vi "Log Trace.vi"(8 "error in (no error)":errorcluster, 10 "Trace.lvclass":refnum<class "Trace.lvclass">, 11 "Tracer in":refnum<class "Tracer.lvclass">) -> (0 "error out":errorcluster, 2 "TraceMessage Out":refnum<class "Trace.lvclass">, 3 "Tracer out":refnum<class "Tracer.lvclass">)   [LabVIEW 2013, in "Tracer.lvclass"]
uses:
  Tracer.lvclass
  TraceMessage/Trace.lvclass
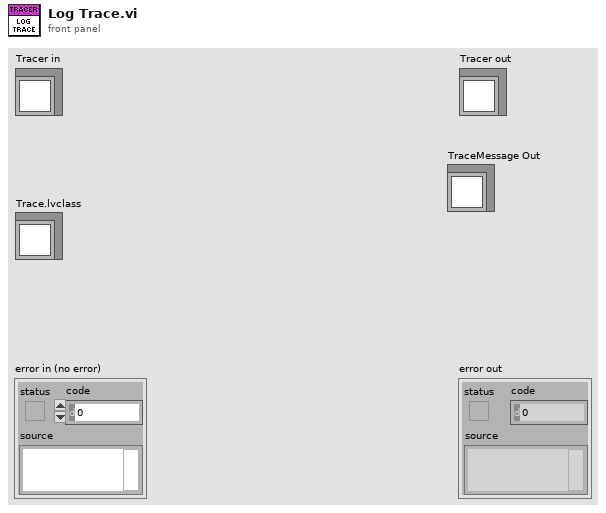
[diagram p1: front panel]
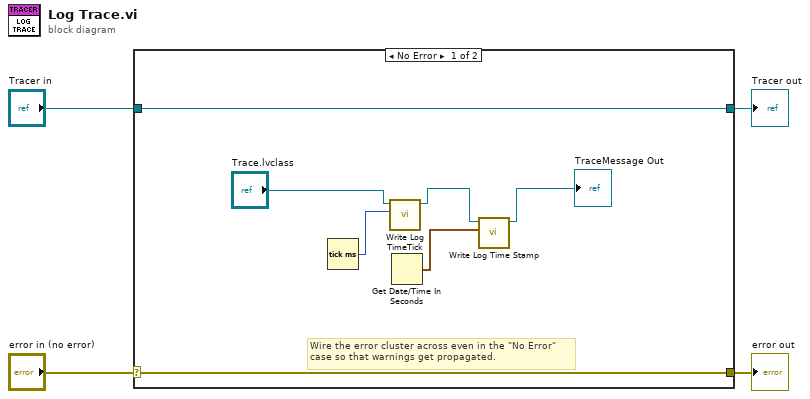
[diagram p0: block diagram]
diagram:
  n1 = case shown="No Error" "error in (no error)" {
    selector: "error in (no error)" -> [w11 w13]
    tunnel: [w11 w13] -> w3
    tunnel: [w10 w12] -> w1
    tunnel: "Tracer in" -> [w10 w12]
    frame No Error {
      # "Wire the error cluster across even in the \"No Error\"\ncase so that warnings get propagated."
      n2 = Tick Count (ms)() -> (millisecond timer value=w9:u32)
      n3 = call-dynamic "Write Log TimeTick.vi"("Trace TimeTick"=w9, "TraceMessage in"="Trace.lvclass") -> ("TraceMessage out"=w7:refnum<class "Trace.lvclass">)  [unwired: 8 in, 1 out]
      n4 = Get Date/Time In Seconds() -> (seconds since 1Jan1904=w5:timestamp)
      n5 = call-dynamic "Write Log Time Stamp.vi"("Log Time Stamp"=w5, "Trace in"=w7) -> ("Trace out"=→"TraceMessage Out":refnum<class "Trace.lvclass">)  [unwired: 8 in, 1 out]
    }
    frame Error {
    }
  }
  "error out" <- w3
  "Tracer out" <- w1
